vi "IMU Serial Read.vi"(3 "Tune bits":u32, 5 "Tune stop bit":u32, 7 "Tune half bit":u32, 8 "Invert Polarity?":bool, 9 "data bits (8)":i32=8 min=5 max=8 step=1, 10 "stop bits (10: 1 bit)":u16(ring)=10 items=["1.0"=10, "1.5"=15, "2.0"=20], 11 "baud rate (230400)":u32=230400) -> ()   [LabVIEW 2021]
uses:
  <vilib>/rvi/Emulation/niFpgaGetClockAttributes.vi
  <vilib>/rvi/Emulation/niFpgaSctlEmulationGetInTimedLoop.vi
  <vilib>/rvi/Emulation/niFpgaEmulationReportErrorSimple.vi
  <vilib>/rvi/eio/common/nirviEmuTemplateMethod_errors.vi
  <vilib>/rvi/Emulation/niFpgaCriticalErrorInLSC.vi
  <vilib>/rvi/Emulation/niFpgaProcessEmulError.vi
  <vilib>/rvi/Emulation/niFpgaEmulationIsFPGAContextNoSignature.vi
  <vilib>/rvi/errors/niFpgaSetErrorForExecOnDevCompSimple.vi
  <vilib>/rvi/eio/common/nirviEmuReportErrorAndStop.vi
  <vilib>/rvi/DataTransferAndStorage/Container/Common/niFpgaContainerGetUniqueNameForEmu.vi
  <vilib>/rvi/FIFO/Fifo_Resource/nirvififoEmulationSetSize.vi
  <vilib>/rvi/FIFO/Fifo_Resource/nirviFifoEmulationQueueMgr.vi
  <instcachedir>/0/nirviFifoEmulationQueueMgr_E5CAEC123FF24DC58D834DCA3CDAA9B5.lvgen/nirviFifoEmulationQueueMgr_E5CAEC123FF24DC58D834DCA3CDAA9B5_001.vi
  <vilib>/rvi/FIFO/Fifo_Resource/nirvififoEmulationDetermineInputValidOut.vi
  <vilib>/rvi/FIFO/Fifo_Resource/nirvififoEmulationCreateLock.vi
  <vilib>/rvi/FIFO/Fifo_Resource/nirvififoEmulationObtainLock.vi
  <vilib>/rvi/FIFO/Fifo_Resource/nirvififoEmulationReleaseLock.vi
  <vilib>/rvi/occurrence/nirviWaitOnOccurrenceBase.vi
  <vilib>/rvi/errors/nirviReportUnexpectedCaseInternalError.vi
  <vilib>/rvi/errors/nirviReportUnexpectedCaseInternalError (U32).vi
  <vilib>/eio/EIONode/EIONode.xnode
  <vilib>/rvi/DataTransferAndStorage/Container/XNode/niFpgaContainer.xnode
  <vilib>/rvi/FIFO/Fifo_Resource/nirvififoEmulationWrite.vi
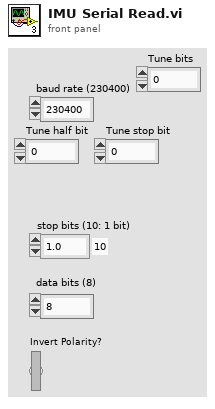
[diagram p1: front panel]
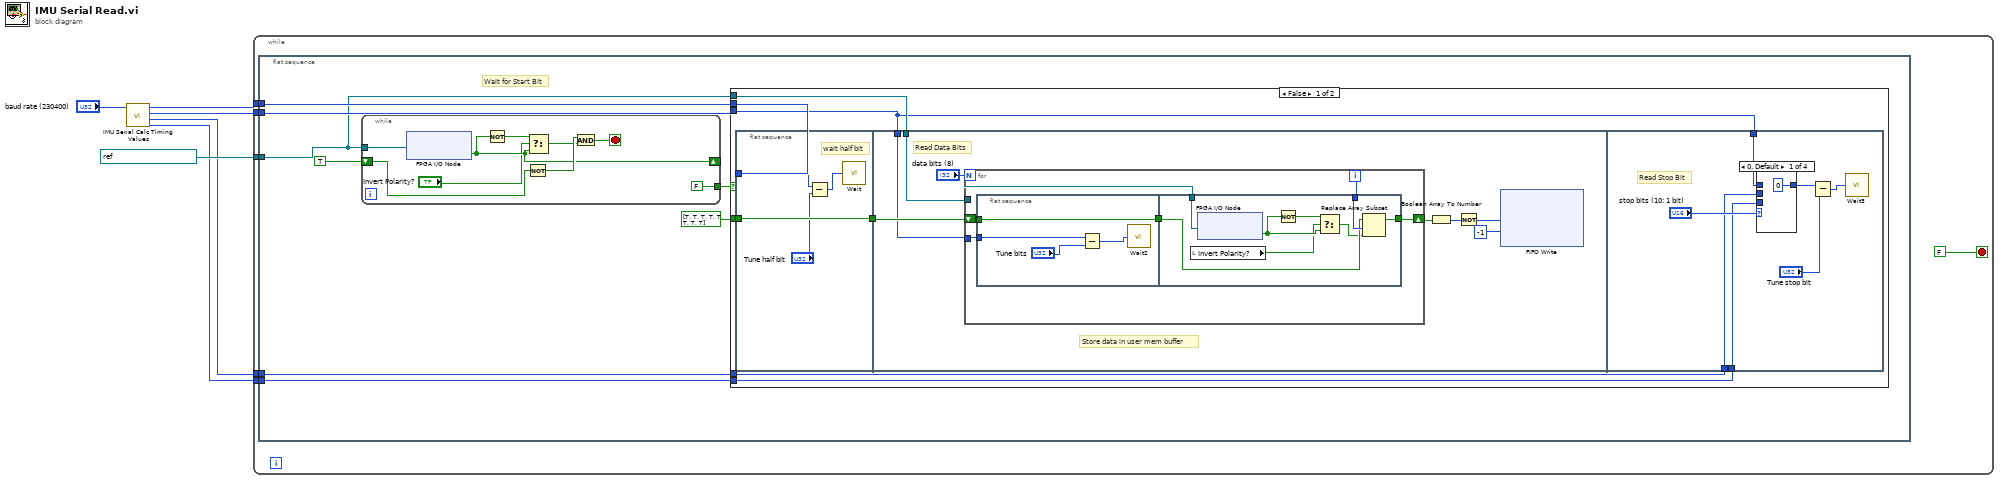
[diagram p0: block diagram]
diagram:
  n1 = call "IMU Serial Calc Timing Values.vi"("baud rate (1000000)"="baud rate (230400)") -> ("Two Bit"=w2:u32, "One and Half Bit"=w3:u32, "One Bit"=w4:u32, "Half Bit"=w5:u32)  [unwired: 3 in]
  n2 = while {
    tunnel: w2 -> [w12]
    tunnel: w3 -> [w11]
    tunnel: w4 -> [w10]
    tunnel: w5 -> [w9]
    tunnel: refnum<k21> "ConnectorA/DIO10" ("Receive") -> [w8]
    stop <- FALSE stop-if-true
    n3 = flat-sequence {
      tunnel: w12 -> [w19]
      tunnel: w11 -> [w18]
      tunnel: w10 -> [w17]
      tunnel: w9 -> [w16]
      tunnel: w8 -> [w13]
      frame #0 {
        # "Wait for Start Bit"
        n4 = while {
          tunnel: [FALSE] -> w15
          shift-right: [w71] -> _
          shift-left: TRUE -> [w76]
          tunnel: w13 -> [w74]
          stop <- w69 stop-if-true
          n5 = xnode "FPGA I/O Node"("FPGA I/O In"=w74) -> ("I/O Item"=w71:bool)  [unwired: 1 out]
          n6 = Not(x=w71) -> (.not. x?=w73:bool)
          n7 = Not(x=w76) -> (.not. x?=w75:bool)
          n8 = Select(t=w73, s="Invert Polarity?", f=w71) -> (s? t:f=w72:bool)
          n9 = And(x=w75, y=w72) -> (x .and. y?=w69:bool)
        }
        n10 = case shown="False" w15 {
          tunnel: bool[] [TRUE, TRUE, TRUE, TRUE, TRUE, TRUE, TRUE, TRUE] -> [w27 _]
          tunnel: w16 -> [w26 _]
          tunnel: w17 -> [w24 _]
          tunnel: w18 -> [w22 _]
          tunnel: w19 -> [w23 _]
          tunnel: w13 -> [w25 _]
          frame False {
            n11 = flat-sequence {
              tunnel: [w31] -> w21
              tunnel: w27 -> [w31]
              tunnel: w26 -> [w30]
              tunnel: w24 -> [w38]
              tunnel: w25 -> [w34]
              tunnel: w21 -> [w39]
              tunnel: w22 -> [w61]
              tunnel: w23 -> [w62]
              tunnel: w24 -> [w63]
              frame #0 {
                # "wait half bit"
                n12 = Subtract(x=w30, y="Tune half bit") -> (x-y=w29:u32)
                n13 = call "Wait"("Count(Ticks)"=w29) -> ()  [unwired: 1 out]
              }
              frame #1 {
                # "Store data in user mem buffer"
                # "Read Data Bits"
                n14 = for {
                  N: "data bits (8)" -> [_]
                  shift-right: [w42] -> w37
                  shift-left: w39 -> [w45]
                  tunnel: w38 -> [w43]
                  tunnel: w34 -> [w40]
                  i -> [w41]
                  n15 = flat-sequence {
                    tunnel: w45 -> [w49]
                    tunnel: [w49] -> w44
                    tunnel: w43 -> [w48]
                    tunnel: w41 -> [w57]
                    tunnel: w44 -> [w56]
                    tunnel: [w55] -> w42
                    tunnel: w40 -> [w54]
                    frame #0 {
                      n16 = Subtract(x=w48, y="Tune bits") -> (x-y=w47:u32)
                      n17 = call "Wait2"("Count(Ticks)"=w47) -> ()  [unwired: 1 out]
                    }
                    frame #1 {
                      n18 = local read "Invert Polarity?"() -> (w50:bool)
                      n19 = xnode "FPGA I/O Node"("FPGA I/O In"=w54) -> ("I/O Item"=w51:bool)  [unwired: 1 out]
                      n20 = Not(x=w51) -> (.not. x?=w53:bool)
                      n21 = Select(t=w53, s=w50, f=w51) -> (s? t:f=w52:bool)
                      n22 = Replace Array Subset(array=w56, new element=w52, index=w57) -> (w55:bool[])
                    }
                  }
                }
                n23 = Boolean Array To Number(Boolean array=w37) -> (number=w36:u8)
                n24 = Not(x=w36) -> (.not. x?=w33:u8)
                n25 = xnode ("FIFO Write")("Element"=w33, "Timeout"=-1) -> ()  [unwired: 1 in, 2 out]
              }
              frame #2 {
                # "Read Stop Bit"
                n26 = case shown="0, Default" "stop bits (10: 1 bit)" {
                  tunnel: w63 -> [_ w66 _ _]
                  tunnel: w61 -> [_ _ w67 _]
                  tunnel: w62 -> [_ _ _ w68]
                  tunnel: [u32 0 ("One Bit") w66 w67 w68] -> w60
                  frame 0, Default {
                  }
                  frame 10 {
                  }
                  frame 15 {
                  }
                  frame 20 {
                  }
                }
                n27 = Subtract(x=w60, y="Tune stop bit") -> (x-y=w59:u32)
                n28 = call "Wait3"("Count(Ticks)"=w59) -> ()  [unwired: 1 out]
              }
            }
          }
          frame True {
          }
        }
      }
    }
  }
